vi "oa_Set Reset True If Parameters Change (1 channel).vi"(7 "reset? (T) in":bool=TRUE, 8 "FIR filter specifications in":T1={"alias rejection (dB)"=120.0, "normalized bandwidth"=0.4536} {"normalized bandwidth" format="%.4f"; "alias rejection (dB)" format="%.2f"}, 9 "interpolation mode in":u16(ring)=1 items=["coerce", "linear", "spline", "FIR filter"], 10 "dr in":dbl=1.0 format="%.2p", 11 "even angle signal in":cluster{"r0":dbl, "dr":dbl, "Y":dbl[]}={"r0"=0.0, "dr"=1.0, "Y"=[]} {"r0" format="%.2p"; "dr" format="%.2p"; "Y" format="%.2f"}) -> (0 "FIR filter specifications out":T1={"alias rejection (dB)"=120.0, "normalized bandwidth"=0.4536} {"normalized bandwidth" format="%.4f"; "alias rejection (dB)" format="%.2f"}, 1 "interpolation mode out":u16(ring)=1 items=["coerce", "linear", "spline", "FIR filter"], 2 "dr out":dbl=1.0 format="%.2p", 3 "even angle signal out":cluster{"r0":dbl, "dr":dbl, "Y":dbl[]}={"r0"=0.0, "dr"=1.0, "Y"=[]} {"r0" format="%.2p"; "dr" format="%.2p"; "Y" format="%.2f"}, 5 "reset? (T) out":bool=TRUE)   [LabVIEW 2017, in "SoundVib_OAUtility.lvlib"]
uses:
  <vilib>/addons/Sound and Vibration/Order Analysis/Utility/SoundVib_OAUtility.lvlib
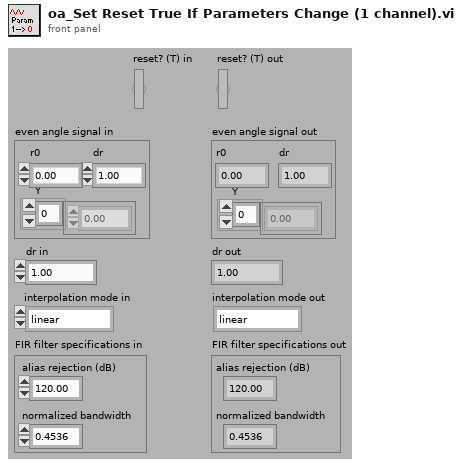
[diagram p1: front panel]
types:
  T1 = cluster{"alias rejection (dB)":dbl, "normalized bandwidth":dbl}
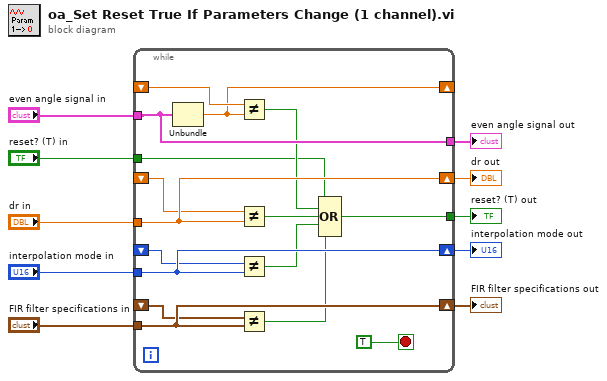
[diagram p0: block diagram]
diagram:
  n1 = while {
    tunnel: "dr in" -> [w25]
    shift-right: [w25] -> w3
    shift-left: _ -> [w24]
    tunnel: "interpolation mode in" -> [w23]
    shift-right: [w23] -> w2
    shift-left: _ -> [w22]
    tunnel: "FIR filter specifications in" -> [w21]
    shift-right: [w21] -> w1
    shift-left: _ -> [w20]
    tunnel: "even angle signal in" -> [w19]
    tunnel: [w19] -> w6
    shift-right: [w17] -> _
    shift-left: _ -> [w18]
    tunnel: "reset? (T) in" -> [w15]
    tunnel: [w11] -> w4
    stop <- TRUE stop-if-true
    n2 = Unbundle(w19) -> ("dr"=w17:dbl)  [unwired: 2 out]
    n3 = Not Equal?(x=w18, y=w17) -> (x != y?=w16:bool)
    n4 = Not Equal?(x=w24, y=w25) -> (x != y?=w14:bool)
    n5 = Not Equal?(x=w22, y=w23) -> (x != y?=w13:bool)
    n6 = Not Equal?(x=w20, y=w21) -> (x != y?=w12:bool)
    n7 = Compound Arithmetic op=OR(w15, w16, w14, w13, w12) -> (w11:bool)
  }
  "even angle signal out" <- w6
  "reset? (T) out" <- w4
  "dr out" <- w3
  "interpolation mode out" <- w2
  "FIR filter specifications out" <- w1
